vi "Target.vi"() -> ()   [LabVIEW 2018]
uses:
  <vilib>/Platform/TimedLoop/XDataNode/timing_clust.ctl
  <vilib>/Platform/TimedLoop/XDataNode/nitl_modes.ctl
  <vilib>/Platform/TimedLoop/XDataNode/wakeup.ctl
  <vilib>/rvi/eio/common/nirviEmuTemplateMethod_errors.vi
  <vilib>/rvi/Emulation/niFpgaGetClockAttributes.vi
  <vilib>/rvi/Emulation/niFpgaSctlEmulationGetInTimedLoop.vi
  <vilib>/rvi/Emulation/niFpgaEmulationReportErrorSimple.vi
  <vilib>/rvi/Emulation/niFpgaProcessEmulError.vi
  <vilib>/rvi/Emulation/niFpgaCriticalErrorInLSC.vi
  <vilib>/eio/EIONode/EIONode.xnode
  <vilib>/Platform/TimedLoop/XDataNode/XDataNode.xnode
  <vilib>/Platform/TimedLoop/XDataNode/XDNodeRunTimeDep.lvlib
panel:
  in  "GEN":bool
  in  "IN1 (K1 to GND)":bool
  in  "IN2 (K2 to VCC)":bool
  in  "Stop_FPGA":bool
  in  "TX_DISABLE":bool
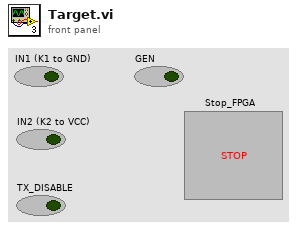
[diagram p1: front panel]
types:
  T1 = typedef "XDNodeRunTimeDep.lvlib/timing_clust.ctl" = cluster{"Expected End [f-1]":u64, "Actual End [f-1]":u64, "Finished Late? [f-1]":bool, "Expected End [i-1]":u64, "Actual End [i-1]":u64, "Finished Late? [i-1]":bool, "Expected Start [i]":u64, "Actual Start [i]":u64, "Expected Start [f]":u64, "Actual Start [f]":u64, "Source Name":string, "Structure Name":string, "Period":i64, "Deadline":i64, "Offset":i64, "Start":i64, "Priority":i32, "Timeout":i32, "Mode":T2, "Wakeup Reason":T3, "Error":errorcluster, "Source Type":string, "Secondary Source Type":string, "Global End Time":u64, "Global Start Time":u64, "Frame Duration":u64, "Iteration Duration":u64, "Assigned CPU":i32, "I/O Scan Engine Mode":u32}
  T2 = typedef "XDNodeRunTimeDep.lvlib/nitl_modes.ctl" = enum32{"No Change", "Process missed periods, maintain original phase", "Discard missed periods, maintain original phase", "Process missed periods, ignore original phase", "Discard missed periods, ignore original phase"}
  T3 = typedef "XDNodeRunTimeDep.lvlib/wakeup.ctl" = enum32{"Normal", "Aborted", "Asynchronous wakeup", "Timing source error", "Timed loop error", "Timeout"}
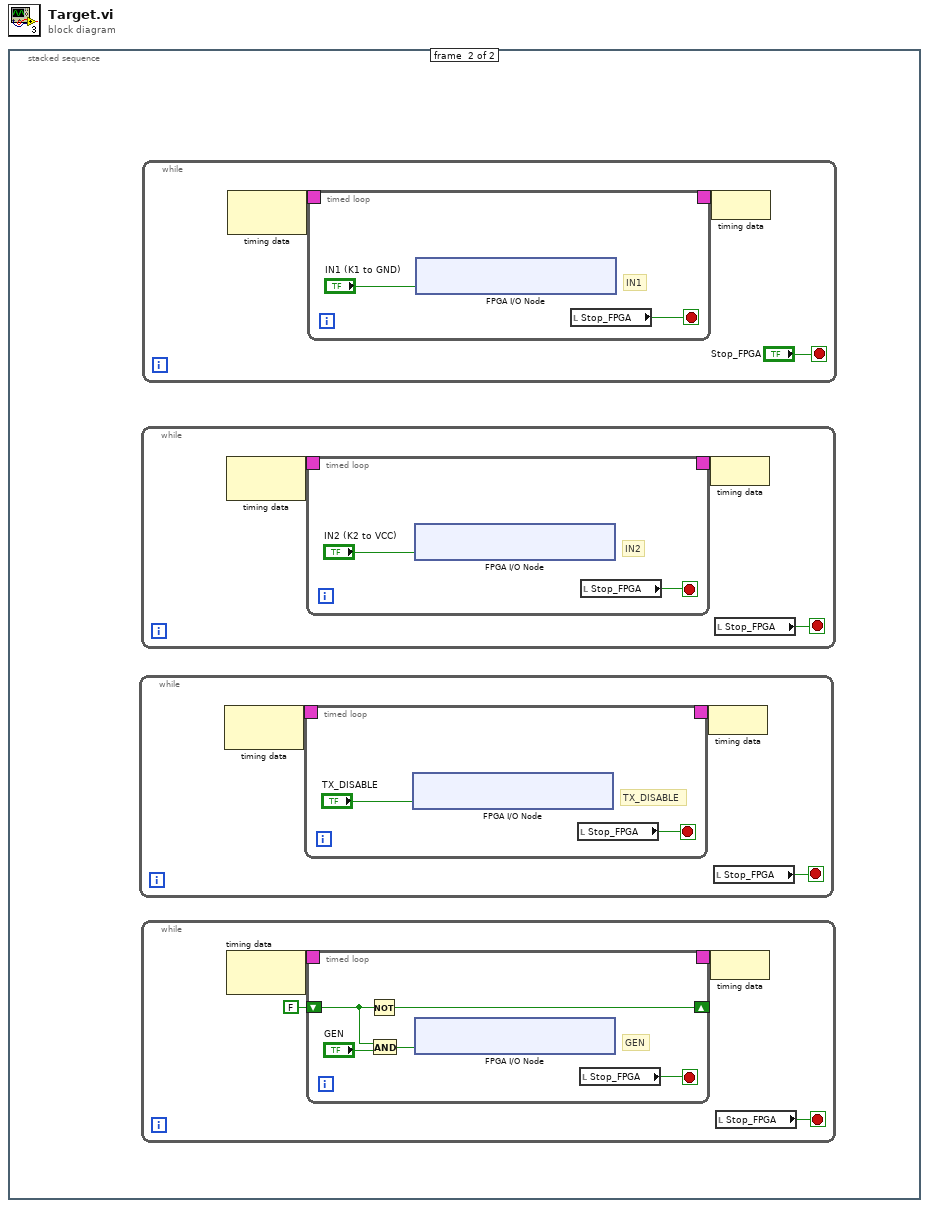
[diagram p0: block diagram]
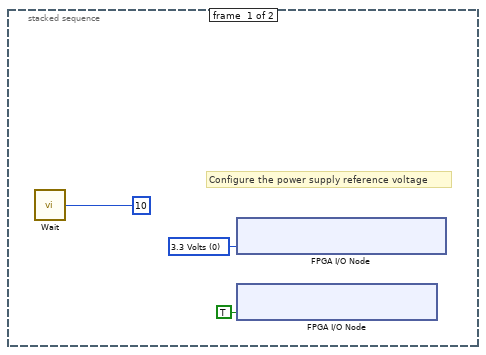
[diagram p2: hidden frame]
diagram:
  n1 = stacked-sequence {
    frame #0 {
      w1 = u8 0 items=["3.3 Volts", "2.5 Volts", "1.8 Volts"] ("Internal Power Supply Voltage")
      # "Configure the power supply reference voltage"
      n2 = call "Wait"("Count(mSec)"=u8 10) -> ()  [unwired: 1 out]
      n3 = xnode "FPGA I/O Node"("IO Module\\Local_Supply_Select"=w1) -> ()  [unwired: 1 in, 1 out]
      n4 = xnode "FPGA I/O Node"("IO Module\\DDCA_DIO0-7_WE"=TRUE ("IO Module\\DDCA_DIO0-7_WE")) -> ()  [unwired: 1 in, 1 out]
    }
    frame #1 {
      n5 = while {
        stop <- w19 stop-if-true
        n6 = node-c288() -> (w18:T1)  [unwired: 1 in]
        n7 = timed-loop {
          timing: w18 -> [_]
          timing-out: [_] -> w17
          stop <- w20 stop-if-true
          # "TX_DISABLE"
          n8 = xnode "FPGA I/O Node"("IO Module\\DDCA_DIO3_Write"="TX_DISABLE") -> ()  [unwired: 1 in, 1 out]
          n9 = local read "Stop_FPGA"() -> (w20:bool)
        }
        n10 = node-c288(w17) -> ()
        n11 = local read "Stop_FPGA"() -> (w19:bool)
      }
      n12 = while {
        stop <- w37 stop-if-true
        n13 = node-c288() -> (w36:T1)  [unwired: 1 in]
        n14 = timed-loop {
          timing: w36 -> [_]
          timing-out: [_] -> w35
          stop <- w38 stop-if-true
          # "IN2"
          n15 = xnode "FPGA I/O Node"("IO Module\\DDCA_DIO1_Write"="IN2 (K2 to VCC)") -> ()  [unwired: 1 in, 1 out]
          n16 = local read "Stop_FPGA"() -> (w38:bool)
        }
        n17 = node-c288(w35) -> ()
        n18 = local read "Stop_FPGA"() -> (w37:bool)
      }
      n19 = while {
        stop <- w7 stop-if-true
        n20 = node-c288() -> (w6:T1)  [unwired: 1 in]
        n21 = timed-loop {
          timing: w6 -> [_]
          timing-out: [_] -> w5
          shift-right: [w8] -> _
          shift-left: FALSE -> [w9]
          stop <- w12 stop-if-true
          # "GEN"
          n22 = Not(x=w9) -> (.not. x?=w8:bool)
          n23 = And(x=w9, y="GEN") -> (x .and. y?=w10:bool)
          n24 = xnode "FPGA I/O Node"("IO Module\\DDCA_DIO7_Write"=w10) -> ()  [unwired: 1 in, 1 out]
          n25 = local read "Stop_FPGA"() -> (w12:bool)
        }
        n26 = node-c288(w5) -> ()
        n27 = local read "Stop_FPGA"() -> (w7:bool)
      }
      n28 = while {
        stop <- "Stop_FPGA" stop-if-true
        n29 = node-c288() -> (w28:T1)  [unwired: 1 in]
        n30 = timed-loop {
          timing: w28 -> [_]
          timing-out: [_] -> w27
          stop <- w29 stop-if-true
          # "IN1"
          n31 = xnode "FPGA I/O Node"("IO Module\\DDCA_DIO0_Write"="IN1 (K1 to GND)") -> ()  [unwired: 1 in, 1 out]
          n32 = local read "Stop_FPGA"() -> (w29:bool)
        }
        n33 = node-c288(w27) -> ()
      }
    }
  }
